vi "PH_BlackBox.ProcCases.vi"(0 "i ref in":refnum<vi>, 1 "selector":string, 2 "Data":T1, 3 "call cluster":T2={"Object"="", "Selector"="", "CallType"=enum."synchronous", "Async Object"="", "Async Selector"="", "Data Descriptor"="", "Data"=[], "Error #"=0, "Expire"=0}, 5 "error in (no error)":errorcluster) -> (14 "i ref out":refnum<vi>, 17 "answer cluster":T2={"Object"="", "Selector"="", "CallType"=enum."synchronous", "Async Object"="", "Async Selector"="", "Data Descriptor"="", "Data"=[], "Error #"=0, "Expire"=0}, 19 "error out":errorcluster)   [LabVIEW 2014, in "PH_BlackBox.lvlib"]
doc: "This method is called by a process from within the default case in the event loop. The methods of a class that are linked to events will be called from THIS method. Add your code here."
uses:
  PH_BlackBox.lvlib
  CSCore/CSSystem/CoreDefs/CoreDefs.call_type.ctl
  CSCore/BaseProcess/BaseProcess.descriptor string definition.ctl
  CSCore/CSSystem/CoreDefs/CoreDefs.rawDataType.ctl
  CSCore/CSSystem/CoreLib/CoreLib.string 2 byte array.vi
  CSCore/CSSystem/CoreLib/CoreLib.byte array 2 short.vi
  CSCore/CSSystem/CoreLib/CoreLib.byte array 2 string.vi
  CSCore/BaseProcess/BaseProcess.lvlib
  PH_Common/PH_Common.lvlib
  CSCore/CAEObj/CAEObj.lvlib
  CSCore/CSSystem/CoreLib/CoreLib.lvlib
  PH_PSDBWriter/PH_PSDBWriter.lvlib
  PH_StatusHandler/PH_StatusHandler.lvlib
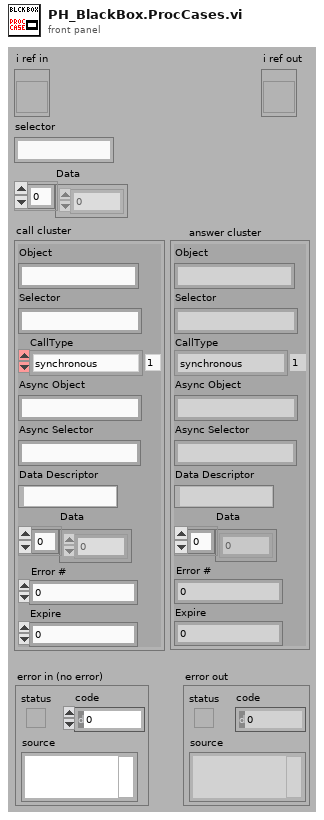
[diagram p1: front panel]
types:
  T1 = typedef "CoreDefs.rawDataType.ctl" = i8[]
  T2 = typedef "CoreDefs.call_type.ctl" = cluster{"Object":string, "Selector":string, "CallType":enum16{"simple", "synchronous", "asynchronous"}, "Async Object":string, "Async Selector":string, "Data Descriptor":T3, "Data":T1, "Error #":i32, "Expire":u32}
  T3 = typedef "BaseProcess.lvlib/BaseProcess.descriptor string definition.ctl" = string
  T4 = typedef "PH_BlackBox.lvlib/PH_BlackBox.i attribute.ctl" = cluster{"BB Remote Controlled?":bool, "GUI Refs":T5, "Position IN":T6, "Position OUT":T6, "BB Remote Controlled by other Instance?":bool, "Recipient":string, "Number":i32, "Caption Move":string, "Caption Out":string, "Caption In":string}
  T5 = typedef "PH_BlackBox.lvlib/PH_BlackBox.GUI Refs.ctl" = cluster{"MOVE IN":refnum<vi>, "MOVE":refnum<vi>, "IN":refnum<vi>, "OUT":refnum<vi>, "REMOTE":refnum<vi>, "GUI-Knob Move":refnum<vi>, "GUI-Knob Move in":refnum<vi>, "POWER ON":refnum<vi>, "Delete":refnum<vi>, "Function Textfield":refnum<vi>}
  T6 = typedef "PH_StatusHandler.lvlib/PH_StatusHandler.Status.ctl" = i16
  T7 = typedef "PH_PSDBWriter.lvlib/PH_PSDBWriter.PHELIX-Subsystems.ctl" = i32
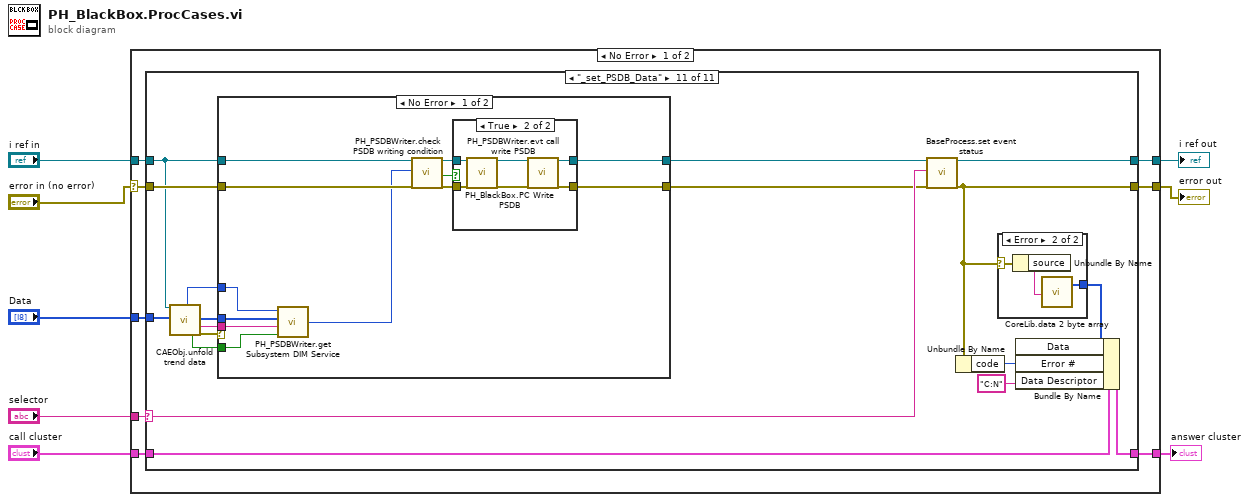
[diagram p0: block diagram]
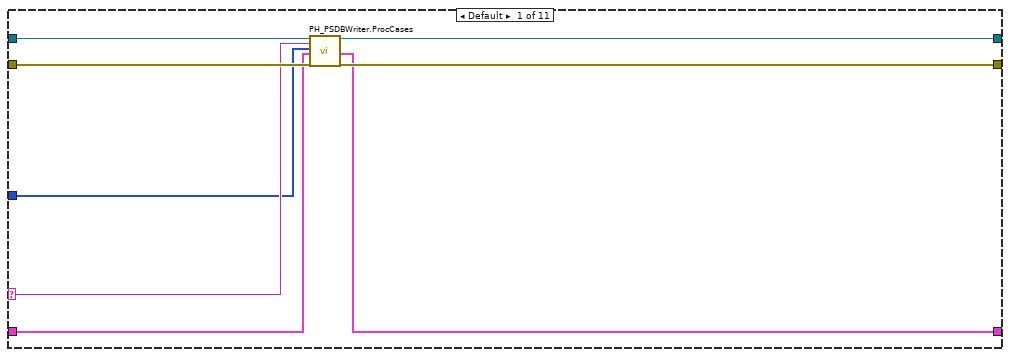
[diagram p2: hidden frame]
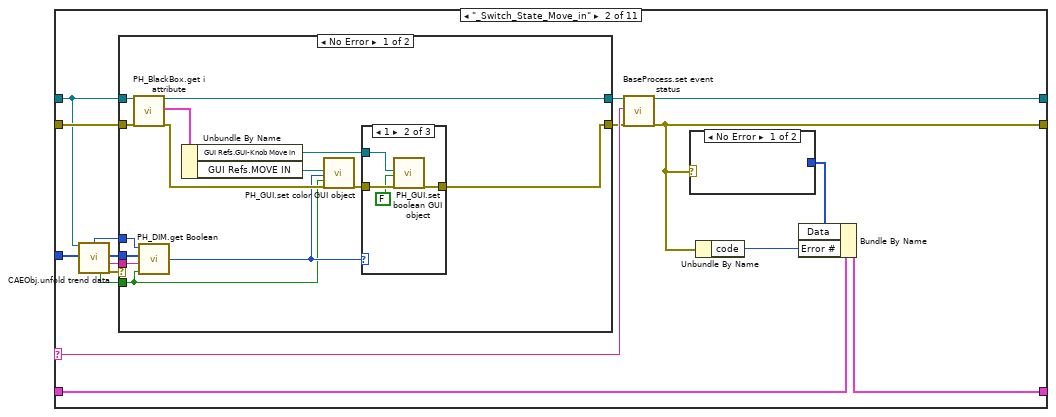
[diagram p3: hidden frame]
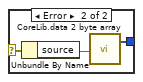
[diagram p4: hidden frame]
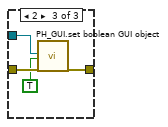
[diagram p6: hidden frame]
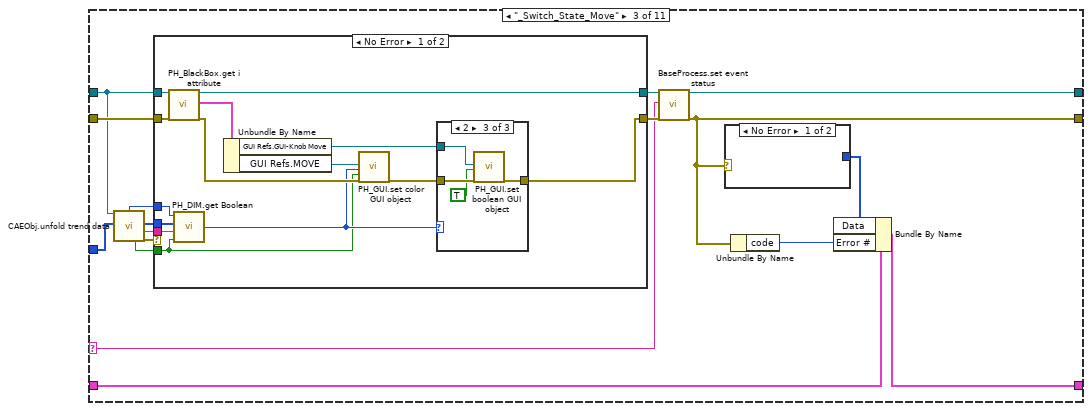
[diagram p8: hidden frame]
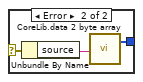
[diagram p9: hidden frame]
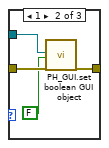
[diagram p11: hidden frame]
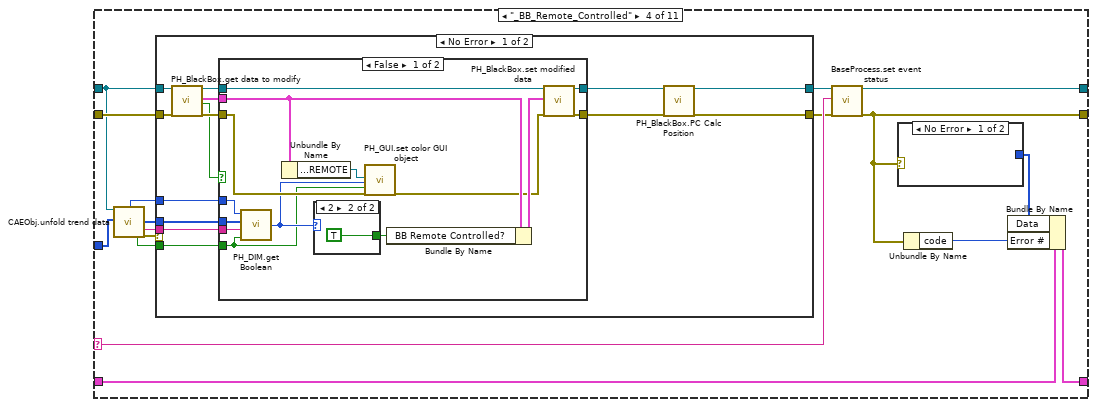
[diagram p13: hidden frame]
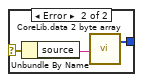
[diagram p14: hidden frame]
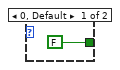
[diagram p15: hidden frame]
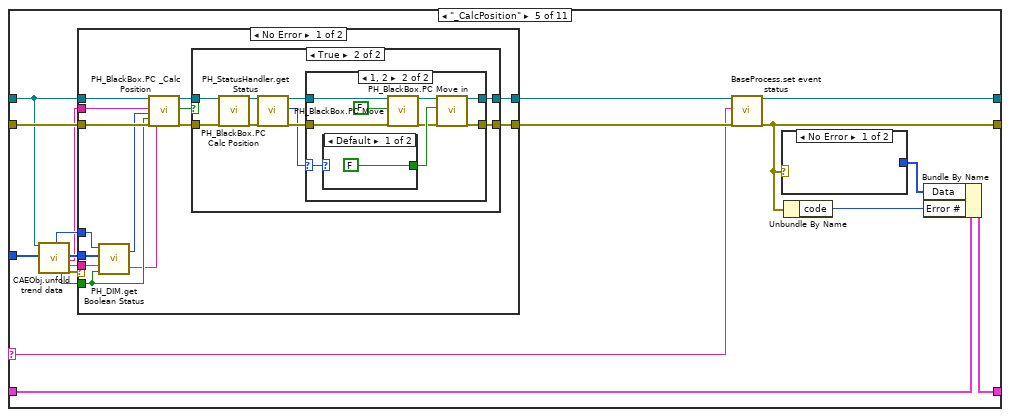
[diagram p18: hidden frame]
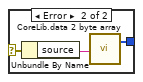
[diagram p19: hidden frame]
diagram:
  n1 = case shown="No Error" "error in (no error)" {
    selector: "error in (no error)" -> [w9 w446]
    tunnel: "selector" -> [w16 _]
    tunnel: [w15 w445] -> w7
    tunnel: "call cluster" -> [w14 w445]
    tunnel: "i ref in" -> [w13 w447]
    tunnel: [w12 w447] -> w4
    tunnel: [w11 w446] -> w3
    tunnel: "Data" -> [w10 _]
    frame No Error {
      n2 = case shown="\"_set_PSDB_Data\"" w16 {
        selector: w16 -> [w19 w31 w74 w121 w172 w232 w272 w324 w344 w386 w411]
        tunnel: w10 -> [w17 w40 w75 w129 w185 w245 _ _ _ _ w407]
        tunnel: w13 -> [w18 w39 w76 w128 w184 w244 w276 w332 w348 w389 w406]
        tunnel: [w24 w28 w71 w115 w174 w233 w270 w327 w355 w383 w413] -> w12
        tunnel: w14 -> [w20 w27 w73 w117 w171 w231 w266 w321 w351 w378 w408]
        tunnel: [w21 w26 w72 w118 w170 w230 w271 w325 w353 w381 w410] -> w15
        tunnel: w9 -> [w23 w41 w77 w131 w186 w246 w277 w333 w346 w390 w418]
        tunnel: [w22 w25 w70 w119 w173 w234 w269 w326 w354 w382 w412] -> w11
        frame Default {
          n3 = call "PH_PSDBWriter.ProcCases.vi"("i ref in"=w18, "selector"=w19, "Data"=w17, "call cluster"=w20, "error in"=w23) -> ("i ref out"=w24:refnum<vi>, "answer cluster"=w21:T2, "error out"=w22:errorcluster)  [unwired: 12 in]
        }
        frame "_Switch_State_Move_in" {
          n4 = call "CAEObj.unfold trend data.vi"("i ref in"=w39, "raw trend data"=w40) -> ("quality"=w34:i32, "no link"=w35:bool, "data"=w37:i8[], "typeDescriptor"=w36:string, "error out"=w38:errorcluster)  [unwired: 9 in, 4 out]
          n5 = case shown="No Error" w38 {
            tunnel: [w55 w69] -> w30
            tunnel: w39 -> [w58 w69]
            tunnel: w41 -> [w57 w68]
            tunnel: [w50 w68] -> w29
            tunnel: w37 -> [w48 _]
            tunnel: w36 -> [w47 _]
            tunnel: w35 -> [w45 _]
            tunnel: w34 -> [w46 _]
            frame No Error {
              n6 = call "PH_BlackBox.get i attribute.vi"("i ref in"=w58, "error in (no error)"=w57) -> ("i ref out"=w55:refnum<vi>, "i attribute"=w56:T4, "error out"=w54:errorcluster)  [unwired: 15 in]
              n7 = call "PH_DIM.get Boolean.vi"("no link"=w45, "typeDescriptor"=w47, "data"=w48, "quality"=w46) -> ("Value"=w49:i32)
              n8 = Unbundle By Name(w56) -> ("GUI Refs.GUI-Knob Move in"=w52:refnum<vi>, "GUI Refs.MOVE IN"=w53:refnum<vi>)
              n9 = call "PH_GUI.set color GUI object.vi"("GUI object Ref"=w53, "State"=w49, "Blinking? (false)"=w45, "error in (no error)"=w54) -> ("error out"=w51:errorcluster)  [unwired: 15 in]
              n10 = case shown="1" w49 {
                tunnel: w52 -> [_ w63 w67]
                tunnel: w51 -> [w59 w62 w66]
                tunnel: [w59 w60 w65] -> w50
                frame 0, Default {
                }
                frame 1 {
                  n11 = call "PH_GUI.set boolean GUI object.vi"("Boolean Knob GUI Ref"=w63, "Value"=FALSE, "error in (no error)"=w62) -> ("error out"=w60:errorcluster)  [unwired: 16 in]
                }
                frame 2 {
                  n12 = call "PH_GUI.set boolean GUI object.vi"("Boolean Knob GUI Ref"=w67, "Value"=TRUE, "error in (no error)"=w66) -> ("error out"=w65:errorcluster)  [unwired: 16 in]
                }
              }
            }
            frame Error {
            }
          }
          n13 = call "BaseProcess.set event status.vi"("i ref in"=w30, "EventStatus"=w31, "error in (no error)"=w29) -> ("i ref out"=w28:refnum<vi>, "error out"=w25:errorcluster)  [unwired: 14 in, 1 out]
          n14 = case shown="No Error" w25 {
            selector: w25 -> [_ w44]
            tunnel: [_ w42] -> w32
            frame No Error {
            }
            frame Error {
              n15 = Unbundle By Name(w44) -> ("source"=w43:string)
              n16 = call-poly "CoreLib.data 2 byte array.vi"("string"=w43) -> ("byteArray out"=w42:T1)  [unwired: 18 in]
            }
          }
          n17 = Unbundle By Name(w25) -> ("code"=w33:i32)
          n18 = Bundle By Name(cluster=w27, "Data"=w32, "Error #"=w33) -> (w26:T2)
        }
        frame "_Switch_State_Move" {
          n19 = call "CAEObj.unfold trend data.vi"("i ref in"=w76, "raw trend data"=w75) -> ("quality"=w82:i32, "no link"=w83:bool, "data"=w85:i8[], "typeDescriptor"=w84:string, "error out"=w86:errorcluster)  [unwired: 9 in, 4 out]
          n20 = case shown="No Error" w86 {
            tunnel: [w100 w114] -> w79
            tunnel: w76 -> [w103 w114]
            tunnel: w77 -> [w102 w113]
            tunnel: [w95 w113] -> w78
            tunnel: w85 -> [w93 _]
            tunnel: w84 -> [w92 _]
            tunnel: w83 -> [w90 _]
            tunnel: w82 -> [w91 _]
            frame No Error {
              n21 = call "PH_BlackBox.get i attribute.vi"("i ref in"=w103, "error in (no error)"=w102) -> ("i ref out"=w100:refnum<vi>, "i attribute"=w101:T4, "error out"=w99:errorcluster)  [unwired: 15 in]
              n22 = call "PH_DIM.get Boolean.vi"("no link"=w90, "typeDescriptor"=w92, "data"=w93, "quality"=w91) -> ("Value"=w94:i32)
              n23 = Unbundle By Name(w101) -> ("GUI Refs.GUI-Knob Move"=w97:refnum<vi>, "GUI Refs.MOVE"=w98:refnum<vi>)
              n24 = call "PH_GUI.set color GUI object.vi"("GUI object Ref"=w98, "State"=w94, "Blinking? (false)"=w90, "error in (no error)"=w99) -> ("error out"=w96:errorcluster)  [unwired: 15 in]
              n25 = case shown="2" w94 {
                tunnel: w97 -> [_ w108 w112]
                tunnel: w96 -> [w104 w107 w111]
                tunnel: [w104 w106 w110] -> w95
                frame 0, Default {
                }
                frame 1 {
                  n26 = call "PH_GUI.set boolean GUI object.vi"("Boolean Knob GUI Ref"=w108, "Value"=FALSE, "error in (no error)"=w107) -> ("error out"=w106:errorcluster)  [unwired: 16 in]
                }
                frame 2 {
                  n27 = call "PH_GUI.set boolean GUI object.vi"("Boolean Knob GUI Ref"=w112, "Value"=TRUE, "error in (no error)"=w111) -> ("error out"=w110:errorcluster)  [unwired: 16 in]
                }
              }
            }
            frame Error {
            }
          }
          n28 = call "BaseProcess.set event status.vi"("i ref in"=w79, "EventStatus"=w74, "error in (no error)"=w78) -> ("i ref out"=w71:refnum<vi>, "error out"=w70:errorcluster)  [unwired: 14 in, 1 out]
          n29 = case shown="No Error" w70 {
            selector: w70 -> [_ w89]
            tunnel: [_ w87] -> w80
            frame No Error {
            }
            frame Error {
              n30 = Unbundle By Name(w89) -> ("source"=w88:string)
              n31 = call-poly "CoreLib.data 2 byte array.vi"("string"=w88) -> ("byteArray out"=w87:T1)  [unwired: 18 in]
            }
          }
          n32 = Unbundle By Name(w70) -> ("code"=w81:i32)
          n33 = Bundle By Name(cluster=w73, "Data"=w80, "Error #"=w81) -> (w72:T2)
        }
        frame "_BB_Remote_Controlled" {
          n34 = call "CAEObj.unfold trend data.vi"("i ref in"=w128, "raw trend data"=w129) -> ("quality"=w126:i32, "no link"=w124:bool, "data"=w125:i8[], "typeDescriptor"=w127:string, "error out"=w130:errorcluster)  [unwired: 9 in, 4 out]
          n35 = case shown="No Error" w130 {
            tunnel: [w135 w168] -> w116
            tunnel: w128 -> [w148 w168]
            tunnel: w131 -> [w147 w167]
            tunnel: [w137 w167] -> w120
            tunnel: w127 -> [w141 _]
            tunnel: w126 -> [w140 _]
            tunnel: w125 -> [w139 _]
            tunnel: w124 -> [w138 _]
            frame No Error {
              n36 = call "PH_BlackBox.get data to modify.vi"("i ref in"=w148, "error in (no error)"=w147) -> ("i ref out"=w145:refnum<vi>, "i attribute"=w143:T4, "timed out"=w142:bool, "error out"=w146:errorcluster)  [unwired: 14 in]
              n37 = case shown="False" w142 {
                tunnel: w146 -> [w162 w165]
                tunnel: w145 -> [w160 w166]
                tunnel: [w159 w166] -> w136
                tunnel: [w158 w165] -> w144
                tunnel: w143 -> [w157 _]
                tunnel: w141 -> [w153 _]
                tunnel: w140 -> [w152 _]
                tunnel: w139 -> [w151 _]
                tunnel: w138 -> [w150 _]
                frame False {
                  n38 = call "PH_DIM.get Boolean.vi"("no link"=w150, "typeDescriptor"=w153, "data"=w151, "quality"=w152) -> ("Value"=w154:i32)
                  n39 = Unbundle By Name(w157) -> ("GUI Refs.REMOTE"=w161:refnum<vi>)
                  n40 = case shown="2" w154 {
                    tunnel: [FALSE TRUE] -> w155
                    frame 0, Default {
                    }
                    frame 2 {
                    }
                  }
                  n41 = call "PH_GUI.set color GUI object.vi"("GUI object Ref"=w161, "State"=w154, "Blinking? (false)"=w150, "error in (no error)"=w162) -> ("error out"=w149:errorcluster)  [unwired: 15 in]
                  n42 = Bundle By Name(cluster=w157, "BB Remote Controlled?"=w155) -> (w156:T4)
                  n43 = call "PH_BlackBox.set modified data.vi"("i ref in"=w160, "i attribute"=w156, "error in (no error)"=w149) -> ("i ref out"=w159:refnum<vi>, "error out"=w158:errorcluster)  [unwired: 15 in]
                }
                frame True {
                }
              }
              n44 = call "PH_BlackBox.PC Calc Position.vi"("i ref in"=w136, "error in (no error)"=w144) -> ("i ref out"=w135:refnum<vi>, "error out"=w137:errorcluster)  [unwired: 16 in]
            }
            frame Error {
            }
          }
          n45 = call "BaseProcess.set event status.vi"("i ref in"=w116, "EventStatus"=w121, "error in (no error)"=w120) -> ("i ref out"=w115:refnum<vi>, "error out"=w119:errorcluster)  [unwired: 14 in, 1 out]
          n46 = case shown="No Error" w119 {
            selector: w119 -> [_ w134]
            tunnel: [_ w132] -> w122
            frame No Error {
            }
            frame Error {
              n47 = Unbundle By Name(w134) -> ("source"=w133:string)
              n48 = call-poly "CoreLib.data 2 byte array.vi"("string"=w133) -> ("byteArray out"=w132:T1)  [unwired: 18 in]
            }
          }
          n49 = Unbundle By Name(w119) -> ("code"=w123:i32)
          n50 = Bundle By Name(cluster=w117, "Data"=w122, "Error #"=w123) -> (w118:T2)
        }
        frame "_CalcPosition" {
          n51 = call "CAEObj.unfold trend data.vi"("i ref in"=w184, "raw trend data"=w185) -> ("quality"=w179:i32, "no link"=w182:bool, "data"=w180:i8[], "serviceName"=w169:string, "typeDescriptor"=w181:string, "error out"=w183:errorcluster)  [unwired: 9 in, 3 out]
          n52 = case shown="No Error" w183 {
            tunnel: [w197 w229] -> w175
            tunnel: w184 -> [w200 w229]
            tunnel: w186 -> [w199 w228]
            tunnel: [w196 w228] -> w176
            tunnel: w181 -> [w203 _]
            tunnel: w182 -> [w191 _]
            tunnel: w180 -> [w202 _]
            tunnel: w179 -> [w201 _]
            tunnel: w169 -> [w194 _]
            frame No Error {
              n53 = call "PH_DIM.get Boolean Status.vi"("no link"=w191, "typeDescriptor"=w203, "data"=w202, "quality"=w201) -> ("further information"=w190:string, "Status"=w193:T6)
              n54 = call "PH_BlackBox.PC _Calc Position.vi"("i ref in"=w200, "serviceName"=w194, "Value"=w193, "No link"=w191, "error in (no error)"=w199, "Tip Strip"=w190) -> ("i ref out"=w195:refnum<vi>, "Status changed?"=w192:bool, "error out"=w198:errorcluster)  [unwired: 11 in]
              n55 = case shown="True" w192 {
                tunnel: w198 -> [w204 w214]
                tunnel: [w205 w212] -> w197
                tunnel: [w204 w210] -> w196
                tunnel: w195 -> [w205 w208]
                frame False {
                }
                frame True {
                  n56 = call "PH_BlackBox.PC Calc Position.vi"("i ref in"=w208, "error in (no error)"=w214) -> ("i ref out"=w207:refnum<vi>, "error out"=w209:errorcluster)  [unwired: 16 in]
                  n57 = call "PH_StatusHandler.get Status.vi"("VI in"=w207, "error in"=w209) -> ("VI out"=w213:refnum<vi>, "Status"=w206:T6, "error out"=w211:errorcluster)  [unwired: 15 in]
                  n58 = case shown="1, 2" w206 {
                    selector: w206 -> [_ w223]
                    tunnel: [w216 w220] -> w212
                    tunnel: [w215 w219] -> w210
                    tunnel: w211 -> [w215 w225]
                    tunnel: w213 -> [w216 w224]
                    frame 0, Default {
                    }
                    frame 1, 2 {
                      n59 = case shown="Default" w223 {
                        tunnel: [FALSE TRUE] -> w221
                        frame Default {
                        }
                        frame 1 {
                        }
                      }
                      n60 = call "PH_BlackBox.PC Move.vi"("i ref in"=w224, "Move?"=FALSE, "error in (no error)"=w225) -> ("i ref out"=w218:refnum<vi>, "error out"=w217:errorcluster)  [unwired: 15 in]
                      n61 = call "PH_BlackBox.PC Move in.vi"("i ref in"=w218, "Move in?"=w221, "error in (no error)"=w217) -> ("i ref out"=w220:refnum<vi>, "error out"=w219:errorcluster)  [unwired: 15 in]
                    }
                  }
                }
              }
            }
            frame Error {
            }
          }
          n62 = call "BaseProcess.set event status.vi"("i ref in"=w175, "EventStatus"=w172, "error in (no error)"=w176) -> ("i ref out"=w174:refnum<vi>, "error out"=w173:errorcluster)  [unwired: 14 in, 1 out]
          n63 = case shown="No Error" w173 {
            selector: w173 -> [_ w189]
            tunnel: [_ w187] -> w177
            frame No Error {
            }
            frame Error {
              n64 = Unbundle By Name(w189) -> ("source"=w188:string)
              n65 = call-poly "CoreLib.data 2 byte array.vi"("string"=w188) -> ("byteArray out"=w187:T1)  [unwired: 18 in]
            }
          }
          n66 = Unbundle By Name(w173) -> ("code"=w178:i32)
          n67 = Bundle By Name(cluster=w171, "Data"=w177, "Error #"=w178) -> (w170:T2)
        }
        frame "_PowerOn" {
          n68 = call "CAEObj.unfold trend data.vi"("i ref in"=w244, "raw trend data"=w245) -> ("quality"=w243:i32, "no link"=w241:bool, "data"=w240:i8[], "typeDescriptor"=w242:string, "error out"=w239:errorcluster)  [unwired: 9 in, 4 out]
          n69 = case shown="No Error" w239 {
            tunnel: [w255 w263] -> w235
            tunnel: w244 -> [w261 w263]
            tunnel: w246 -> [w260 w262]
            tunnel: [w256 w262] -> w236
            tunnel: w243 -> [w254 _]
            tunnel: w242 -> [w253 _]
            tunnel: w241 -> [w250 _]
            tunnel: w240 -> [w252 _]
            frame No Error {
              n70 = call "PH_BlackBox.get i attribute.vi"("i ref in"=w261, "error in (no error)"=w260) -> ("i ref out"=w255:refnum<vi>, "i attribute"=w258:T4, "error out"=w259:errorcluster)  [unwired: 15 in]
              n71 = call "PH_DIM.get Boolean.vi"("no link"=w250, "typeDescriptor"=w253, "data"=w252, "quality"=w254) -> ("Value"=w251:i32)
              n72 = Unbundle By Name(w258) -> ("GUI Refs.POWER ON"=w257:refnum<vi>)
              n73 = call "PH_GUI.set color GUI object.vi"("GUI object Ref"=w257, "State"=w251, "Blinking? (false)"=w250, "error in (no error)"=w259) -> ("error out"=w256:errorcluster)  [unwired: 15 in]
            }
            frame Error {
            }
          }
          n74 = call "BaseProcess.set event status.vi"("i ref in"=w235, "EventStatus"=w232, "error in (no error)"=w236) -> ("i ref out"=w233:refnum<vi>, "error out"=w234:errorcluster)  [unwired: 14 in, 1 out]
          n75 = case shown="No Error" w234 {
            selector: w234 -> [_ w249]
            tunnel: [_ w247] -> w237
            frame No Error {
            }
            frame Error {
              n76 = Unbundle By Name(w249) -> ("source"=w248:string)
              n77 = call-poly "CoreLib.data 2 byte array.vi"("string"=w248) -> ("byteArray out"=w247:T1)  [unwired: 18 in]
            }
          }
          n78 = Unbundle By Name(w234) -> ("code"=w238:i32)
          n79 = Bundle By Name(cluster=w231, "Data"=w237, "Error #"=w238) -> (w230:T2)
        }
        frame "Control Remote" {
          n80 = Unbundle By Name(w266) -> ("Data"=w268:T1)
          n81 = call-poly "CoreLib.byte array 2 data.vi"("byteArray"=w268) -> ("i16"=w267:i16, "error out"=w265:errorcluster)  [unwired: 16 in, 1 out]
          n82 = Greater Than 0?(x=w267) -> (x > 0?=w264:bool)
          n83 = case shown="No Error" w265 {
            tunnel: [w282 w318] -> w270
            tunnel: w276 -> [w289 w318]
            tunnel: w277 -> [w288 w317]
            tunnel: [w284 w317] -> w269
            tunnel: w264 -> [w286 _]
            frame No Error {
              n84 = call "PH_BlackBox.get data to modify.vi"("i ref in"=w289, "error in (no error)"=w288) -> ("i ref out"=w283:refnum<vi>, "i attribute"=w287:T4, "timed out"=w281:bool, "error out"=w285:errorcluster)  [unwired: 14 in]
              n85 = case shown="False" w281 {
                tunnel: w287 -> [w292 _]
                tunnel: w286 -> [w291 _]
                tunnel: w285 -> [w297 w315]
                tunnel: [w295 w315] -> w284
                tunnel: w283 -> [w294 w316]
                tunnel: [w293 w316] -> w282
                frame False {
                  n86 = Unbundle By Name(w292) -> ("GUI Refs.GUI-Knob Move"=w300:refnum<vi>, "GUI Refs.GUI-Knob Move in"=w301:refnum<vi>, "GUI Refs.Delete"=w296:refnum<vi>)
                  n87 = case shown="True" w291 {
                    tunnel: [0 2] -> w298
                    frame False {
                    }
                    frame True {
                    }
                  }
                  n88 = Build Array(w300, w301, w296) -> (w299:refnum<vi>[])
                  n89 = for {
                    shift-right: [w307] -> w302
                    shift-left: w297 -> [w309]
                    tunnel: w299 -> [w306] mode=indexing
                    tunnel: w298 -> [w305]
                    n90 = Not A Number/Path/Refnum?(number/path/refnum=w306) -> (NaN/Path/Refnum?=w308:bool)
                    n91 = case shown="False" w308 {
                      tunnel: w306 -> [w313 _]
                      tunnel: w309 -> [w312 w314]
                      tunnel: [w311 w314] -> w307
                      tunnel: w305 -> [w310 _]
                      frame False {
                        n92 = property class="Bool"(reference=w313, error in=w312, "Disabled"=w310) -> (error out=w311:errorcluster)  [unwired: 1 out]
                      }
                      frame True {
                      }
                    }
                  }
                  n93 = Bundle By Name(cluster=w292, "BB Remote Controlled by other Instance?"=w291) -> (w290:T4)
                  n94 = call "PH_BlackBox.set modified data.vi"("i ref in"=w294, "i attribute"=w290, "error in (no error)"=w302) -> ("i ref out"=w293:refnum<vi>, "error out"=w295:errorcluster)  [unwired: 15 in]
                }
                frame True {
                }
              }
            }
            frame Error {
            }
          }
          n95 = call "BaseProcess.set event status.vi"("i ref in"=w270, "EventStatus"=w272, "error in (no error)"=w269) -> ("error out"=w273:errorcluster)  [unwired: 14 in, 2 out]
          n96 = case shown="No Error" w273 {
            selector: w273 -> [_ w280]
            tunnel: [_ w278] -> w274
            frame No Error {
            }
            frame Error {
              n97 = Unbundle By Name(w280) -> ("source"=w279:string)
              n98 = call-poly "CoreLib.data 2 byte array.vi"("string"=w279) -> ("byteArray out"=w278:T1)  [unwired: 18 in]
            }
          }
          n99 = Unbundle By Name(w273) -> ("code"=w275:i32)
          n100 = Bundle By Name(cluster=w266, "Data"=w274, "Error #"=w275) -> (w271:T2)
        }
        frame "SetDirection" {
          n101 = Unbundle By Name(w321) -> ("Data"=w322:T1)
          n102 = call-poly "CoreLib.byte array 2 data.vi"("byteArray"=w322) -> ("i16"=w323:i16, "error out"=w320:errorcluster)  [unwired: 16 in, 1 out]
          n103 = Greater Than 0?(x=w323) -> (x > 0?=w319:bool)
          n104 = case shown="No Error" w320 {
            tunnel: [w341 w343] -> w329
            tunnel: [w340 w342] -> w328
            tunnel: w332 -> [w339 w343]
            tunnel: w333 -> [w338 w342]
            tunnel: w319 -> [w337 _]
            frame No Error {
              n105 = call "PH_BlackBox.PC Move in.vi"("i ref in"=w339, "Move in?"=w337, "error in (no error)"=w338) -> ("i ref out"=w341:refnum<vi>, "error out"=w340:errorcluster)  [unwired: 15 in]
            }
            frame Error {
            }
          }
          n106 = call "BaseProcess.set event status.vi"("i ref in"=w329, "EventStatus"=w324, "error in (no error)"=w328) -> ("i ref out"=w327:refnum<vi>, "error out"=w326:errorcluster)  [unwired: 14 in, 1 out]
          n107 = case shown="No Error" w326 {
            selector: w326 -> [_ w336]
            tunnel: [_ w334] -> w330
            frame No Error {
            }
            frame Error {
              n108 = Unbundle By Name(w336) -> ("source"=w335:string)
              n109 = call-poly "CoreLib.data 2 byte array.vi"("string"=w335) -> ("byteArray out"=w334:T1)  [unwired: 18 in]
            }
          }
          n110 = Unbundle By Name(w326) -> ("code"=w331:i32)
          n111 = Bundle By Name(cluster=w321, "Data"=w330, "Error #"=w331) -> (w325:T2)
        }
        frame "Set Function Textfield" {
          n112 = Unbundle By Name(w351) -> ("Data"=w352:T1)
          n113 = call-poly "CoreLib.byte array 2 data.vi"("byteArray"=w352) -> ("string"=w349:string, "error out"=w350:errorcluster)  [unwired: 16 in, 1 out]
          n114 = case shown="No Error" w350 {
            tunnel: [w364 w372] -> w347
            tunnel: w348 -> [w366 w372]
            tunnel: w346 -> [w365 w371]
            tunnel: [w362 w370] -> w345
            tunnel: w344 -> [_ w369]
            tunnel: w349 -> [w359 _]
            frame No Error {
              n115 = call "PH_BlackBox.get i attribute.vi"("i ref in"=w366, "error in (no error)"=w365) -> ("i ref out"=w364:refnum<vi>, "i attribute"=w361:T4, "error out"=w363:errorcluster)  [unwired: 15 in]
              n116 = Unbundle By Name(w361) -> ("GUI Refs.Function Textfield"=w360:refnum<vi>)
              n117 = case shown="Default" w359 {
                tunnel: [TRUE FALSE] -> w358
                frame Default {
                }
                frame "", "N/A" {
                }
              }
              n118 = call "PH_GUI.set string GUI object.vi"("Visible (True)"=w358, "GUI object Ref"=w360, "Text"=w359, "error in"=w363) -> ("error out"=w362:errorcluster)  [unwired: 15 in]
            }
            frame Error {
              n119 = call "CoreLib.set data type mismatch.vi"("error in (no error)"=w371, "error source"=w369) -> ("error out"=w370:errorcluster)  [unwired: 17 in]
            }
          }
          n120 = call "BaseProcess.set event status.vi"("i ref in"=w347, "EventStatus"=w344, "error in (no error)"=w345) -> ("i ref out"=w355:refnum<vi>, "error out"=w354:errorcluster)  [unwired: 14 in, 1 out]
          n121 = case shown="No Error" w354 {
            selector: w354 -> [_ w375]
            tunnel: [_ w373] -> w356
            frame No Error {
            }
            frame Error {
              n122 = Unbundle By Name(w375) -> ("source"=w374:string)
              n123 = call-poly "CoreLib.data 2 byte array.vi"("string"=w374) -> ("byteArray out"=w373:T1)  [unwired: 18 in]
            }
          }
          n124 = Unbundle By Name(w354) -> ("code"=w357:i32)
          n125 = Bundle By Name(cluster=w351, "Data"=w356, "Error #"=w357) -> (w353:T2)
        }
        frame "Move" {
          n126 = Unbundle By Name(w378) -> ("Data"=w379:T1)
          n127 = call-poly "CoreLib.byte array 2 data.vi"("byteArray"=w379) -> ("i16"=w380:i16, "error out"=w376:errorcluster)  [unwired: 16 in, 1 out]
          n128 = Greater Than 0?(x=w380) -> (x > 0?=w377:bool)
          n129 = case shown="No Error" w376 {
            tunnel: [w398 w400] -> w384
            tunnel: [w397 w399] -> w385
            tunnel: w389 -> [w396 w400]
            tunnel: w390 -> [w395 w399]
            tunnel: w377 -> [w394 _]
            frame No Error {
              n130 = call "PH_BlackBox.PC Move.vi"("i ref in"=w396, "Move?"=w394, "error in (no error)"=w395) -> ("i ref out"=w398:refnum<vi>, "error out"=w397:errorcluster)  [unwired: 15 in]
            }
            frame Error {
            }
          }
          n131 = call "BaseProcess.set event status.vi"("i ref in"=w384, "EventStatus"=w386, "error in (no error)"=w385) -> ("i ref out"=w383:refnum<vi>, "error out"=w382:errorcluster)  [unwired: 14 in, 1 out]
          n132 = case shown="No Error" w382 {
            selector: w382 -> [_ w393]
            tunnel: [_ w391] -> w387
            frame No Error {
            }
            frame Error {
              n133 = Unbundle By Name(w393) -> ("source"=w392:string)
              n134 = call-poly "CoreLib.data 2 byte array.vi"("string"=w392) -> ("byteArray out"=w391:T1)  [unwired: 18 in]
            }
          }
          n135 = Unbundle By Name(w382) -> ("code"=w388:i32)
          n136 = Bundle By Name(cluster=w378, "Data"=w387, "Error #"=w388) -> (w381:T2)
        }
        frame "_set_PSDB_Data" {
          n137 = call "CAEObj.unfold trend data.vi"("i ref in"=w406, "raw trend data"=w407) -> ("quality"=w401:i32, "no link"=w404:bool, "data"=w402:i8[], "typeDescriptor"=w403:string, "error out"=w405:errorcluster)  [unwired: 9 in, 4 out]
          n138 = case shown="No Error" w405 {
            tunnel: w418 -> [w430 w440]
            tunnel: [w429 w439] -> w414
            tunnel: [w428 w440] -> w409
            tunnel: w406 -> [w426 w439]
            tunnel: w404 -> [w420 _]
            tunnel: w403 -> [w422 _]
            tunnel: w402 -> [w423 _]
            tunnel: w401 -> [w421 _]
            frame No Error {
              n139 = call "PH_PSDBWriter.get Subsystem DIM Service.vi"("no link"=w420, "typeDescriptor"=w422, "data"=w423, "quality"=w421) -> ("PHELIX Subsystems"=w419:T7)
              n140 = call "PH_PSDBWriter.check PSDB writing condition.vi"("i ref in"=w426, "wanted Subsystem"=w419, "error IO"=w430) -> ("i ref out"=w425:refnum<vi>, "write PSDB?"=w424:bool, "error out"=w427:errorcluster)  [unwired: 14 in]
              n141 = case shown="True" w424 {
                tunnel: w427 -> [w431 w438]
                tunnel: [w432 w435] -> w429
                tunnel: [w431 w433] -> w428
                tunnel: w425 -> [w432 w437]
                frame False {
                }
                frame True {
                  n142 = call "PH_BlackBox.PC Write PSDB.vi"("i ref in"=w437, "error IO"=w438) -> ("i ref out"=w436:refnum<vi>, "error out"=w434:errorcluster)  [unwired: 16 in]
                  n143 = call "PH_PSDBWriter.evt call write PSDB.vi"("i ref in"=w436, "error in (no error)"=w434) -> ("i ref out"=w435:refnum<vi>, "error out"=w433:errorcluster)  [unwired: 16 in]
                }
              }
            }
            frame Error {
            }
          }
          n144 = call "BaseProcess.set event status.vi"("i ref in"=w414, "EventStatus"=w411, "error in (no error)"=w409) -> ("i ref out"=w413:refnum<vi>, "error out"=w412:errorcluster)  [unwired: 14 in, 1 out]
          n145 = Unbundle By Name(w412) -> ("code"=w417:i32)
          n146 = case shown="Error" w412 {
            selector: w412 -> [_ w444]
            tunnel: [T1 [] ("byteArray out") w442] -> w415
            frame No Error {
            }
            frame Error {
              n147 = Unbundle By Name(w444) -> ("source"=w443:string)
              n148 = call-poly "CoreLib.data 2 byte array.vi"("string"=w443) -> ("byteArray out"=w442:T1)  [unwired: 18 in]
            }
          }
          n149 = Bundle By Name(cluster=w408, "Data"=w415, "Error #"=w417, "Data Descriptor"="C:N") -> (w410:T2)
        }
      }
    }
    frame Error {
    }
  }
  "answer cluster" <- w7
  "i ref out" <- w4
  "error out" <- w3
